vi "Alligator Dataset Information Window.vi"() -> ()   [LabVIEW 2021, in "AlliGator Dataset Information Window.lvlib"]
doc: "Window displaying the dataset information extracted from internal variables and settings."
uses:
  AlliGator Dataset Information Window.lvlib
panel:
  out "File Information":string
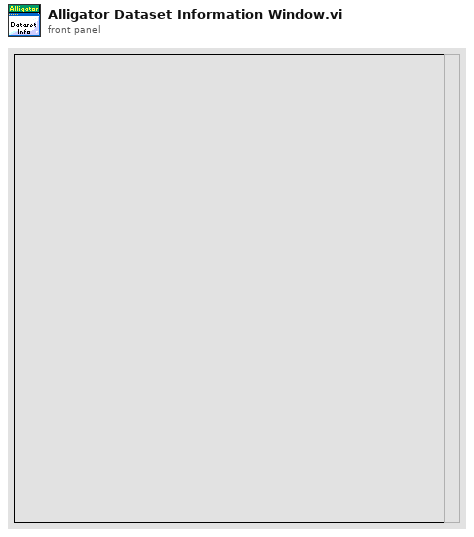
[diagram p1: front panel]
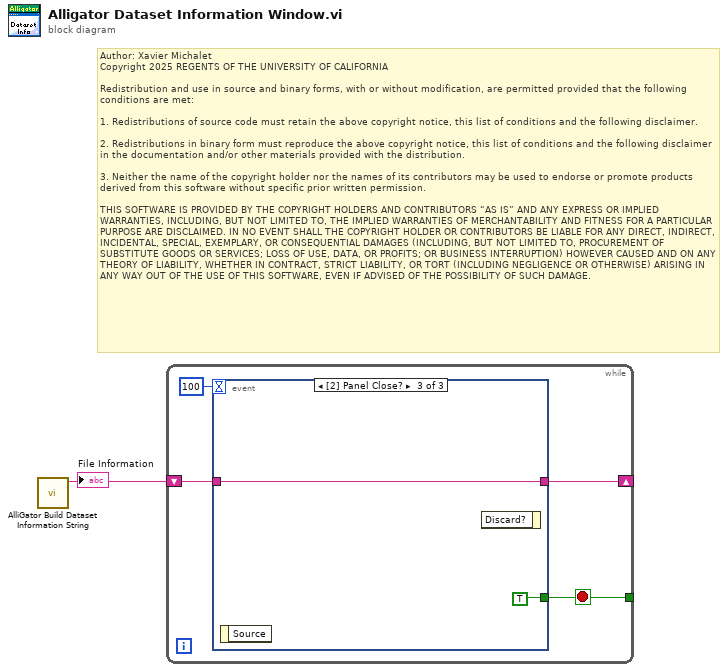
[diagram p0: block diagram]
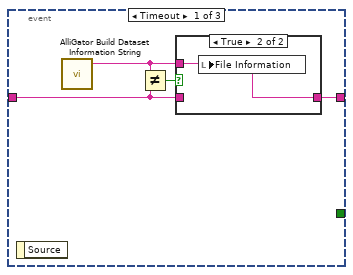
[diagram p2: hidden frame]
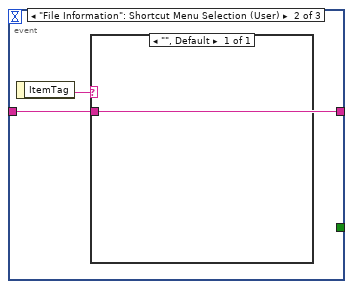
[diagram p4: hidden frame]
diagram:
  # "Author: Xavier Michalet\nCopyright 2025 REGENTS OF THE UNIVERSITY OF CALIFORNIA\n\nRedistribution and use in source and binary forms, with or without modification, are permitted provided that the following conditions are met:\n\n1. Redistributions of source code must retain the above copyright notice, this list of conditions and the following disclaimer.\n\n2. Redistributions in binary form must reproduce the above copyright notice, this list of conditions and the following disclaimer in the documentation and/or other materials provided with the distribution.\n\n3. Neither the name of the copyright holder nor the names of its contributors may be used to endorse or promote products derived from this software without specific prior written permission.\n\nTHIS SOFTWARE IS PROVIDED BY THE COPYRIGHT HOLDERS AND CONTRIBUTORS “AS IS” AND ANY EXPRESS OR IMPLIED WARRANTIES, INCLUDING, BUT NOT LIMITED TO, THE IMPLIED WARRANTIES OF MERCHANTABILITY AND FITNESS FOR A PARTICULAR PURPOSE ARE DISCLAIMED. IN NO EVENT SHALL THE COPYRIGHT HOLDER OR CONTRIBUTORS BE LIABLE FOR ANY DIRECT, INDIRECT, INCIDENTAL, SPECIAL, EXEMPLARY, OR CONSEQUENTIAL DAMAGES (INCLUDING, BUT NOT LIMITED TO, PROCUREMENT OF SUBSTITUTE GOODS OR SERVICES; LOSS OF USE, DATA, OR PROFITS; OR BUSINESS INTERRUPTION) HOWEVER CAUSED AND ON ANY THEORY OF LIABILITY, WHETHER IN CONTRACT, STRICT LIABILITY, OR TORT (INCLUDING NEGLIGENCE OR OTHERWISE) ARISING IN ANY WAY OUT OF THE USE OF THIS SOFTWARE, EVEN IF ADVISED OF THE POSSIBILITY OF SUCH DAMAGE."
  n1 = call "AlliGator Build Dataset Information String.vi"() -> ("Dataset Information String"=w1:string)  [unwired: 11 in]
  "File Information" <- w1
  n2 = while {
    shift-right: [w3] -> _
    shift-left: w1 -> [w4]
    tunnel: [w2] -> _
    stop <- w2 stop-if-true
    n3 = event shown="[2] Panel Close?" {
      selector: _ -> [_ _ _]
      dyn-events: _ -> [_ _ _]
      timeout: 100 -> [_ _ _]
      tunnel: w4 -> [w8 w12 w14]
      tunnel: [w7 w12 w14] -> w3
      tunnel: [_ _ TRUE] -> w2
      event Timeout {
        n4 = event-data() -> ()  [unwired: 1 in, 1 out]
        n5 = call "AlliGator Build Dataset Information String.vi"() -> ("Dataset Information String"=w6:string)  [unwired: 11 in]
        n6 = Not Equal?(x=w6, y=w8) -> (x != y?=w9:bool)
        n7 = case shown="True" w9 {
          tunnel: w6 -> [_ w11]
          tunnel: w8 -> [w10 _]
          tunnel: [w10 w11] -> w7
          frame False {
          }
          frame True {
            n8 = local write "File Information"(w11) -> ()
          }
        }
      }
      event "File Information": Shortcut Menu Selection (User) {
        n9 = event-data() -> ("ItemTag"=w13:string)  [unwired: 1 in]
        n10 = case shown="\"\", Default" w13 {
          tunnel: w12 -> [_]
          frame "", Default {
          }
        }
      }
      event Panel Close? {
        n11 = event-data() -> ()  [unwired: 1 in, 1 out]
        n12 = event-data() -> ()  [unwired: 2 in, 1 out]
      }
    }
  }
